vi "Update Chamber Status.vi"(8 "error in (no error)":errorcluster) -> (0 "error out":errorcluster)   [LabVIEW 2015, in "Thermal Chamber Controller_DQMH.lvlib"]
doc: "Request the Thermal Chamber Controller to Update the Chamber Status. \n\n_____\nCreated using Delacor QMH Event Scripter 1.0.0.50.\n____\nDelacor QMH Thermal Chamber Examples 4.0.0.21\nCopyright (c) 2018, Delacor"
uses:
  Thermal Chamber Controller_DQMH.lvlib
  Update Chamber Status Argument--cluster.ctl
  Heater State--enum.ctl
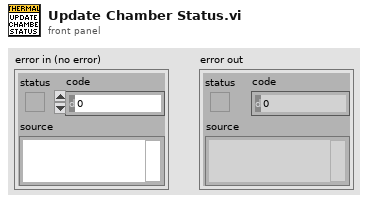
[diagram p1: front panel]
types:
  T1 = typedef "Thermal Chamber Controller_DQMH.lvlib/Update Chamber Status Argument--cluster.ctl" = cluster{"Temperature Set Point":dbl, "Temperature Ramp Rate":dbl, "Heater State":T2, "Actual Temperature":dbl}
  T2 = typedef "Thermal Chamber Controller_DQMH.lvlib/Heater State--enum.ctl" = enum16{"Heater Enabled", "Heater Disabled"}
  T3 = typedef "Thermal Chamber Controller_DQMH.lvlib/Request Events--cluster.ctl" = cluster{"Stop Module":refnum<user-event>, "Show Panel":refnum<user-event>, "Hide Panel":refnum<user-event>, "Get Module Execution Status":refnum<user-event>, "Show Diagram":refnum<user-event>, "Update Set Point":refnum<user-event>, "Update Ramp Rate":refnum<user-event>, "Update Heater State":refnum<user-event>, "Update Chamber Status":refnum<user-event>, "Request and Wait for Status":refnum<user-event>}
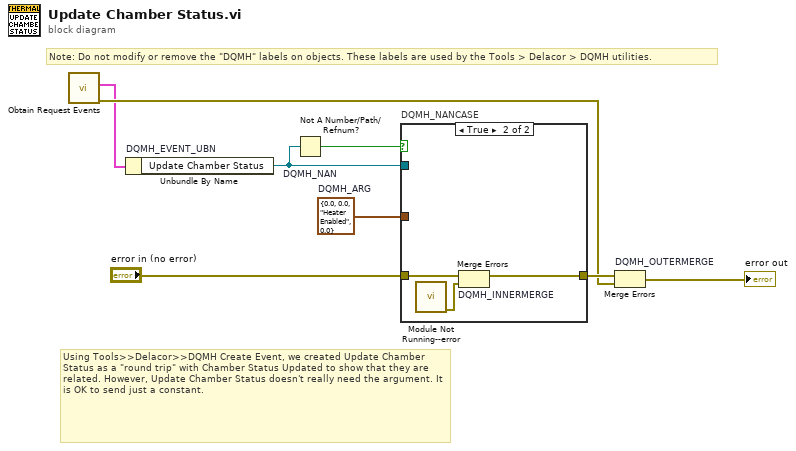
[diagram p0: block diagram]
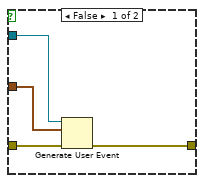
[diagram p2: hidden frame]
diagram:
  w1 = T1 {"Temperature Set Point"=0.0, "Temperature Ramp Rate"=0.0, "Heater State"=enum."Heater Enabled", "Actual Temperature"=0.0}  # DQMH_ARG
  # "Using Tools>>Delacor>>DQMH Create Event, we created Update Chamber Status as a \"round trip\" with Chamber Status Updated to show that they are related. However, Update Chamber Status doesn't really need the argument. It is OK to send just a constant."
  # "Note: Do not modify or remove the \"DQMH\" labels on objects. These labels are used by the Tools > Delacor > DQMH utilities."
  n1 = call "Obtain Request Events.vi"() -> ("error out"=w3:errorcluster, "Thermal Chamber Controller_DQMH Request Events"=w2:T3)  [unwired: 10 in]
  n2 = Unbundle By Name "DQMH_EVENT_UBN"(w2) -> ("Update Chamber Status"=w4:refnum<user-event>)
  n3 = Not A Number/Path/Refnum? "DQMH_NAN"(number/path/refnum=w4) -> (NaN/Path/Refnum?=w5:bool)
  n4 = case "DQMH_NANCASE" shown="True" w5 {
    tunnel: "error in (no error)" -> [w12 w15]
    tunnel: [w11 w14] -> w6
    tunnel: w4 -> [w10 _]
    tunnel: w1 -> [w9 _]
    frame False {
      n5 = Generate User Event(user event=w10, event data cluster=w9, error in=w12) -> (error out=w11:errorcluster)  [unwired: 1 in, 1 out]
    }
    frame True {
      n6 = call "Module Not Running--error.vi"() -> ("error out"=w13:errorcluster)  [unwired: 11 in]
      n7 = Merge Errors "DQMH_INNERMERGE"(w15, w13) -> (w14:errorcluster)
    }
  }
  n8 = Merge Errors "DQMH_OUTERMERGE"(w6, w3) -> (→"error out":errorcluster)
